vi "사칙연산(배열).vi"() -> ()   [LabVIEW 2020]
panel:
  out "SUM X":dbl
  out "X/Y":dbl[](array[numeric])
  out "X*Y":dbl[](array[numeric])
  out "X-Y":dbl[](array[numeric])
  out "X+Y":dbl[](array[numeric])
  out "SUM Y":dbl
  in  "Y":dbl[](array[numeric])
  in  "X":dbl[](array[numeric])
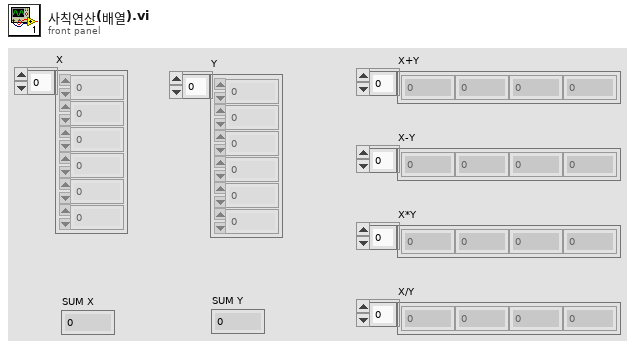
[diagram p1: front panel]
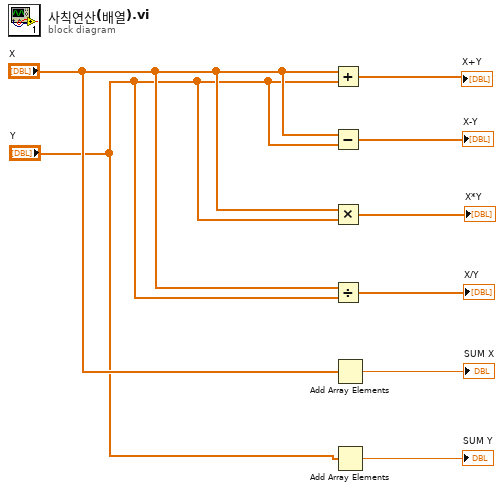
[diagram p0: block diagram]
diagram:
  n1 = Add(x="X", y="Y") -> (x+y=→"X+Y":dbl[])
  n2 = Subtract(x="X", y="Y") -> (x-y=→"X-Y":dbl[])
  n3 = Multiply(x="X", y="Y") -> (x*y=→"X*Y":dbl[])
  n4 = Divide(x="X", y="Y") -> (x/y=→"X/Y":dbl[])
  n5 = Add Array Elements(numeric array="X") -> (sum=→"SUM X":dbl)
  n6 = Add Array Elements(numeric array="Y") -> (sum=→"SUM Y":dbl)
